vi "T1.vi"(2 "Sampling Frequency":dbl=100000000.0 format="%.2e", 3 "Frequency":dbl format="%.2f", 4 "Line Code":string="11001101011") -> (0 "NumberOfSamplesPerBit":i32=26, 1 "Binary Waveform":dbl[](array[numeric]) format="%.2f")   [LabVIEW 2012]
panel:
  out "Waveform Graph":dbl[](graph)
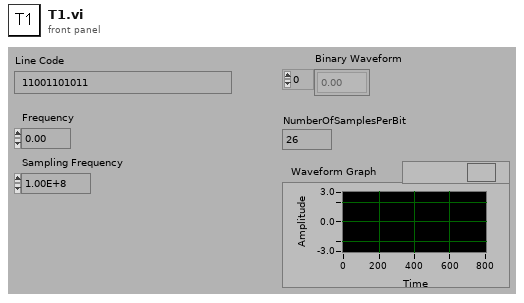
[diagram p1: front panel]
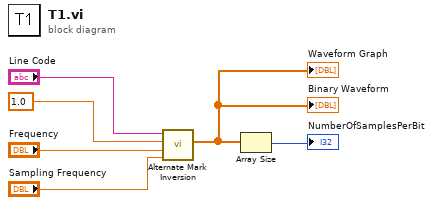
[diagram p0: block diagram]
diagram:
  n1 = call "Alternate Mark Inversion.vi"("Sampling Frequency"="Sampling Frequency", "Frequency"="Frequency", "Amplitude"=1.0 ("Binary1 Level"), "Line Code"="Line Code") -> ("Signal"=w1:dbl[])  [unwired: 1 in, 3 out]
  "Binary Waveform" <- w1
  "Waveform Graph" <- w1
  n2 = Array Size(array=w1) -> (size(s)=→"NumberOfSamplesPerBit":i32)
